vi "Create Slave Instance.vi"   [LabVIEW 2020, in "Modbus Slave.lvclass"]
doc: "Creates a serial or TCP Modbus slave instance. The Modbus slave instance you create includes a daemon. Daemon is a background process that responds to requests from Modbus master instances. You must manually select the polymorphic instance to use."
uses:
  <vilib>/Modbus/slave/Modbus Slave.lvclass
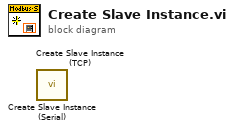
[diagram p0: block diagram]
diagram:
  n1 = call <vilib>:"Create Slave Instance (Serial).vi"() -> ()  [unwired: 10 in, 2 out]
  n2 = call <vilib>:"Create Slave Instance (TCP).vi"() -> ()  [unwired: 10 in, 2 out]
